vi "ep12_for_loop.vi"() -> ()   [LabVIEW 2019]
panel:
  out "led0":bool
  out "led1":bool
  out "Array 2":i32[](array[numeric])
  out "Array":i32[](array[numeric])
  out "Numeric 2":i32
  out "Numeric":i32
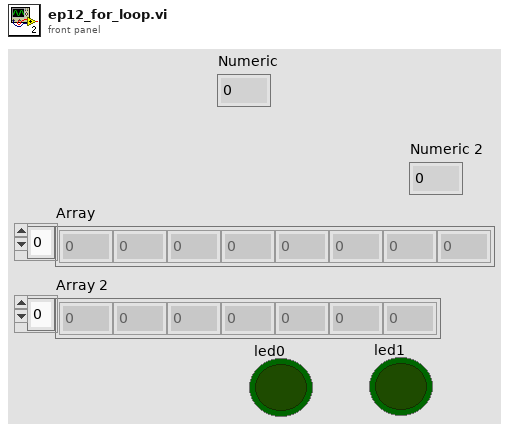
[diagram p1: front panel]
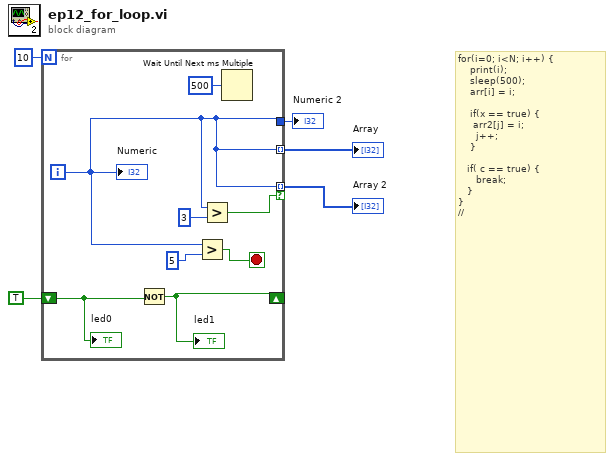
[diagram p0: block diagram]
diagram:
  # "for(i=0; i<N; i++) {\n    print(i);\n    sleep(500); \n    arr[i] = i;\n   \n    if(x == true) {\n     arr2[j] = i;\n      j++;\n    }\n\n   if( c == true) {\n      break;\n   }\n}\n//"
  n1 = for {
    N: 10 -> [_]
    tunnel: [w9] -> w4
    tunnel: [w9] -> w3 mode=indexing
    tunnel: [w9] -> w2 mode=indexing if=w12
    shift-right: [w7] -> _
    shift-left: TRUE -> [w6]
    i -> [w9]
    stop <- w8 stop-if-true
    n2 = Not(x=w6) -> (.not. x?=w7:bool)
    "led1" <- w7
    n3 = Greater?(x=w9, y=5) -> (0:w8:bool)
    n4 = Greater?(x=w9, y=3) -> (0:w12:bool)
    n5 = Wait Until Next ms Multiple(millisecond multiple=u32 500) -> ()  [unwired: 1 out]
    "Numeric" <- w9
    "led0" <- w6
  }
  "Numeric 2" <- w4
  "Array" <- w3
  "Array 2" <- w2
